vi "InvPendSfbTrking_277.vi"() -> ()   [LabVIEW 2016]
uses:
  <vilib>/Analysis/Matrix/Datatypes/RealMatrix.ctl
  <vilib>/Simulation/Scripting/Companion Diagram/SimConfigNode/SimParams.ctl
  <vilib>/Simulation/Scripting/Companion Diagram/SimConfigNode/_simSolvers.ctl
  <vilib>/Simulation/Implementation/Shared/SIMSCR Execution Mode.ctl
  <vilib>/Platform/TimedLoop/XDataNode/timing_clust.ctl
  <vilib>/Platform/TimedLoop/XDataNode/nitl_modes.ctl
  <vilib>/Platform/TimedLoop/XDataNode/wakeup.ctl
  <vilib>/Simulation/Param Hierarchy/Typedefs/SIMPH Param Control Actions.ctl
  <vilib>/Simulation/Implementation/Shared/NILVSim_ParamChanged.vi
  <vilib>/Simulation/Implementation/Shared/NILVSim_FinishedLate.vi
  <vilib>/Simulation/Implementation/Shared/NILVSIM_BeginStep.vi
  <vilib>/Simulation/Utility/Implementation/NILVSim Collector.llb/SIM Collector (scalar).vi
  <vilib>/Simulation/Utility/Implementation/SIM Halt.vi
  <vilib>/Simulation/DataSources/Implementation/NILVSim Sine Wave.llb/SIM Sine Wave (scalar).vi
  <vilib>/Simulation/DiscreteLinear/Implementation/NILVSim Discrete State Space Buffered.llb/SIM Discrete State Space Distributor (SISO).vi
  <vilib>/Simulation/DiscreteLinear/Implementation/NILVSim Discrete State Space Buffered.llb/SIM Discrete State Space Collector (SISO).vi
  <vilib>/Analysis/baseanly.llb/A x B.vi
  <vilib>/Analysis/baseanly.llb/A x Vector.vi
  <vilib>/Simulation/DiscreteLinear/Implementation/NILVSim Discrete Delay.llb/NILVSim Discrete Delay Buffered Distributor (vector).vi
  <vilib>/Simulation/Nonlinear/Implementation/NILVSim Saturation.llb/SIM Saturation (scalar).vi
  <vilib>/Simulation/DiscreteLinear/Implementation/NILVSim Discrete Delay.llb/NILVSim Discrete Delay Buffered Collector (vector).vi
  <vilib>/Simulation/Implementation/Shared/NILVSim_Manager.vi
  <vilib>/Utility/error.llb/Clear Errors.vi
  <vilib>/Simulation/Implementation/Shared/NILVSim_FinalizeModel.vi
  <vilib>/Simulation/Utility/Implementation/NILVSim Collector.llb/NILVSim Collector core (scalar).vi
  <vilib>/Simulation/Implementation/Shared/SIM Unbundle Sim Info.vi
  <vilib>/Simulation/Implementation/Shared/SIMSH Read Queue.vi
  <vilib>/Simulation/Implementation/Shared/NILVSim_Initialize.vi
  <vilib>/Simulation/Utility/Implementation/NILVSim Get Time and IsAcceptedStep.vi
  SubVI/CommandDuty.vi
  <vilib>/Simulation/Implementation/Shared/NILVSim_GetModelError.vi
  <vilib>/Simulation/Implementation/Shared/SIM Bundle Sim Info.vi
  <vilib>/Simulation/Scripting/Companion Diagram/SimConfigNode/SimDog.xnode
  <vilib>/Platform/TimedLoop/XDataNode/XDataNode.xnode
  <vilib>/Simulation/Implementation/XNodeFramework/SimXNode/SimX.xnode
  <vilib>/Analysis/NI_AALBase.lvlib
  <vilib>/Simulation/DiscreteLinear/Implementation/NILVSim Discrete Delay.llb/SIM Discrete Delay Buffered (vector).vi
  <vilib>/Simulation/DiscreteLinear/Implementation/NILVSim Discrete State Space Buffered.llb/SIM Discrete State Space Buffered (SISO).vi
  <vilib>/Platform/TimedLoop/XDataNode/XDNodeRunTimeDep.lvlib
  <vilib>/Simulation/Implementation/Shared/NI_SIM_Implementation.lvlib
  <vilib>/Analysis/Matrix/NI_Matrix.lvlib
panel:
  in  "Tab Control":T1(tab)
  out "Reference r and Output y":cluster{dbl, dbl}(graph)
  out "Control input u":dbl(graph)
  in  "Final Time (s)":dbl=10.0
  in  "Run Control":bool
  in  "K":T2=[[4.67, 70.57]]
  out "y_hat vs y":cluster{"Result":dbl, dbl}(graph)
  in  "Pc":T2=[[0.0, 2.15]]
  in  "Pa":T2=[[1.0012, 0.0117], [0.016, 1.0001]]
  in  "Pb":dbl[](array[numeric])=[0.1281, 0.0001]
  in  "L":dbl[](array[numeric])=[2.925, 0.279]
  in  "Km":T2=[[4.67, 70.57]]
  out "error out":errorcluster
  out "Counter Value":i32
  # "Control Settings"
  # "InvPend Model"
  # "Control Parameters"
  # "Hint: You don't need to do anything in this page"
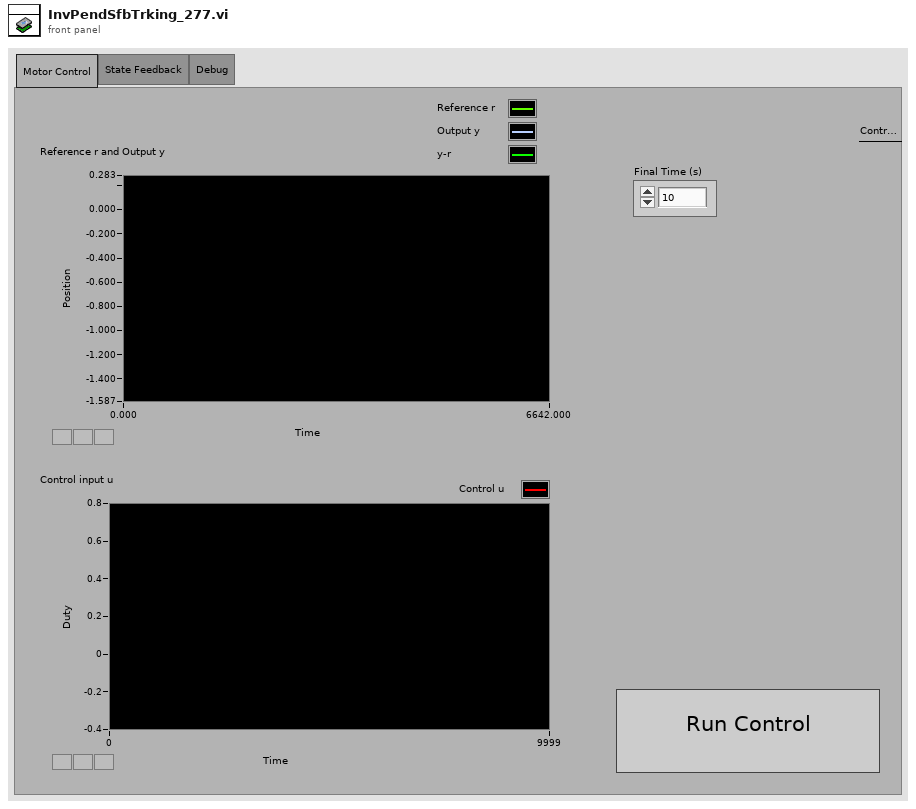
[diagram p1: front panel]
types:
  T1 = enum32{"Motor Control", "State Feedback", "Debug"}
  T2 = typedef "NI_Matrix.lvlib/RealMatrix.ctl" = dbl[][]
  T3 = typedef "SIMSCR Execution Mode.ctl" = enum16{"Simulate to Completion", "Single Time-Step Simulation (Fixed Step Only)"}
  T4 = typedef "XDNodeRunTimeDep.lvlib/timing_clust.ctl" = cluster{"Expected End [f-1]":u64, "Actual End [f-1]":u64, "Finished Late? [f-1]":bool, "Expected End [i-1]":u64, "Actual End [i-1]":u64, "Finished Late? [i-1]":bool, "Expected Start [i]":u64, "Actual Start [i]":u64, "Expected Start [f]":u64, "Actual Start [f]":u64, "Source Name":string, "Structure Name":string, "Period":i64, "Deadline":i64, "Offset":i64, "Start":i64, "Priority":i32, "Timeout":i32, "Mode":T5, "Wakeup Reason":T6, "Error":errorcluster, "Source Type":string, "Secondary Source Type":string, "Global End Time":u64, "Global Start Time":u64, "Frame Duration":u64, "Iteration Duration":u64, "Assigned CPU":i32, "I/O Scan Engine Mode":u32}
  T5 = typedef "XDNodeRunTimeDep.lvlib/nitl_modes.ctl" = enum32{"No Change", "Process missed periods, maintain original phase", "Discard missed periods, maintain original phase", "Process missed periods, ignore original phase", "Discard missed periods, ignore original phase"}
  T6 = typedef "XDNodeRunTimeDep.lvlib/wakeup.ctl" = enum32{"Normal", "Aborted", "Asynchronous wakeup", "Timing source error", "Timed loop error", "Timeout"}
  T7 = typedef "SIMPH Param Control Actions.ctl" = enum16{"get params", "set params"}
  T8 = typedef "SimParams.ctl" = cluster{"Initial Time (s)":dbl, "Final Time (s)":dbl, "Step Size (s)":dbl, "ODE Solver":T9, "Minimum Step Size (s)":dbl, "Maximum Step Size (s)":dbl, "Relative Tolerance":dbl, "Absolute Tolerance":dbl, "Software Timing":bool, "Initial Step Size (s)":dbl, "Automatic Fixed Step Size?":bool, "Automatic Discrete Step Size?":bool, "Discrete Step Size (s)":dbl, "Calculate using Time Step":bool, "Solver Wired?":bool, "Prev.Frm.Expected End":u64, "Prev.Frm.Actual End":u64, "Prev.Frm.Finished Late?":bool, "Prev.Iter.Expected End":u64, "Prev.Iter.Actual End":u64, "Prev.Iter.Finished Late?":bool, "Expected Iteration Start":u64, "Actual Iteration Start":u64, "Expected Frame Start":u64, "Actual Frame Start":u64, "Source Name":string, "Name":string, "Period":i64, "Deadline":i64, "Offset":i64, "Start":i64, "Priority":i32, "Timeout":i32, "Processor":i32, "Mode":enum32{"No Change", "Process missed periods, maintain original phase", "Discard missed periods, maintain original phase", "Process missed periods, ignore original phase", "Discard missed periods, ignore original phase"}, "Wakeup reason":enum32{"Normal", "Aborted", "Asynchronous wakeup", "Timing source error", "Timed loop error", "Timeout"}, "Error":errorcluster, "Source Type":string, "Secondary Source Type":string, "Global End Time":u64, "Global Start Time":u64, "Full Solver Reset":bool, "Execution Mode":T3, "Nan/Inf Check":bool, "Custom Solver Library":string, "Solver Is Variable":bool, "custom solver name":string, "Signal Collection Decimation":u32}
  T9 = typedef "_simSolvers.ctl" = enum16{"Runge-Kutta 1 (Euler)", "Runge-Kutta 2", "Runge-Kutta 3", "Runge-Kutta 4", "Runge-Kutta 23 (variable)", "Runge-Kutta 45 (variable)", "BDF (variable)", "Adams-Moulton (variable)", "Rosenbrock (variable)", "Discrete States Only", "SDIRK 4 (variable)", "Radau 5 (variable)", "Radau 9 (variable)", "Radau 13 (variable)", "Radau [Variable Order] (variable)", "Gear's Method (variable)", "Linearizer", "State Query", "Trim Eval", "Custom Solver"}
  T10 = typedef "PWM.lvlib/PWM Reference.ctl" = cluster{"myRIO Reference":T11, "PWM Channels Enum":T15, "PWM Configuration":T16}
  T11 = typedef "myRIO Generic Hardware Reference.ctl" = cluster{"myRIO Model":T12, "myRIO Hardware Reference":T13}
  T12 = typedef "Hardware Version Enum.ctl" = enum16{"Unknown", "myRIO-1900", "myRIO-1950", "roboRIO", "NI ELVIS RIO CM"}
  T13 = typedef "myRIO v1.0 Reference.ctl" = cluster{"Generic FPGA Reference":T14, "Allow multiple opens":bool}
  T14 = typedef "Generic FPGA Reference.ctl" = refnum<k20>
  T15 = typedef "PWM Channels Enum.ctl" = enum16{"Not Connected", "C/PWM0", "C/PWM1", "A/PWM0", "A/PWM1", "A/PWM2", "B/PWM0", "B/PWM1", "B/PWM2", "PWM/PWM0", "PWM/PWM1", "PWM/PWM2", "PWM/PWM3", "PWM/PWM4", "PWM/PWM5", "PWM/PWM6", "PWM/PWM7", "PWM/PWM8", "PWM/PWM9"}
  T16 = typedef "PWM.lvlib/PWM Configuration.ctl" = cluster{"Frequency":dbl, "Duty Cycle":dbl}
  T17 = typedef "Encoder.lvlib/Encoder Reference.ctl" = cluster{"myRIO Reference":T11, "Encoder Channels Enum":T18}
  T18 = typedef "Encoder Channels Enum.ctl" = enum16{"Not Connected", "C/ENC0", "C/ENC1", "A/ENC", "B/ENC", "DIO/ENC0", "DIO/ENC1", "DIO/ENC2", "DIO/ENC3", "DIO/ENC4"}
  T19 = typedef "DIO.lvlib/DIO Reference.ctl" = cluster{"myRIO Reference":T11, "DIO Channels List":T20}
  T20 = typedef "DIO Channels List.ctl" = T21[]
  T21 = typedef "DIO Channels Enum.ctl" = enum16{"Not Connected", "C/DIO0", "C/DIO1", "C/DIO2", "C/DIO3", "C/DIO4", "C/DIO5", "C/DIO6", "C/DIO7", "A/DIO0", "A/DIO1", "A/DIO2", "A/DIO3", "A/DIO4", "A/DIO5", "A/DIO6", "A/DIO7", "A/DIO8", "A/DIO9", "A/DIO10", "A/DIO11", "A/DIO12", "A/DIO13", "A/DIO14", "A/DIO15", "B/DIO0", "B/DIO1", "B/DIO2", "B/DIO3", "B/DIO4", "B/DIO5", "B/DIO6", "B/DIO7", "B/DIO8", "B/DIO9", "B/DIO10", "B/DIO11", "B/DIO12", "B/DIO13", "B/DIO14", "B/DIO15", "LED0", "LED1", "LED2", "LED3", "Button0", "DIO/DIO0", "DIO/DIO1", "DIO/DIO2", "DIO/DIO3", "DIO/DIO4", "DIO/DIO5", "DIO/DIO6", "DIO/DIO7", "DIO/DIO8", "DIO/DIO9", "SPI/CS0", "SPI/CS1", "SPI/CS2", "SPI/CS3", "LED RADIO (Green)", "LED RADIO (Red)", "LED COMM (Green)", "LED COMM (Red)", "LED MODE (Green)", "LED MODE (Red)"}
  T22 = cluster{"PWM0":T10, "PWM1":T10, "Encoder":T17, "En":T19}
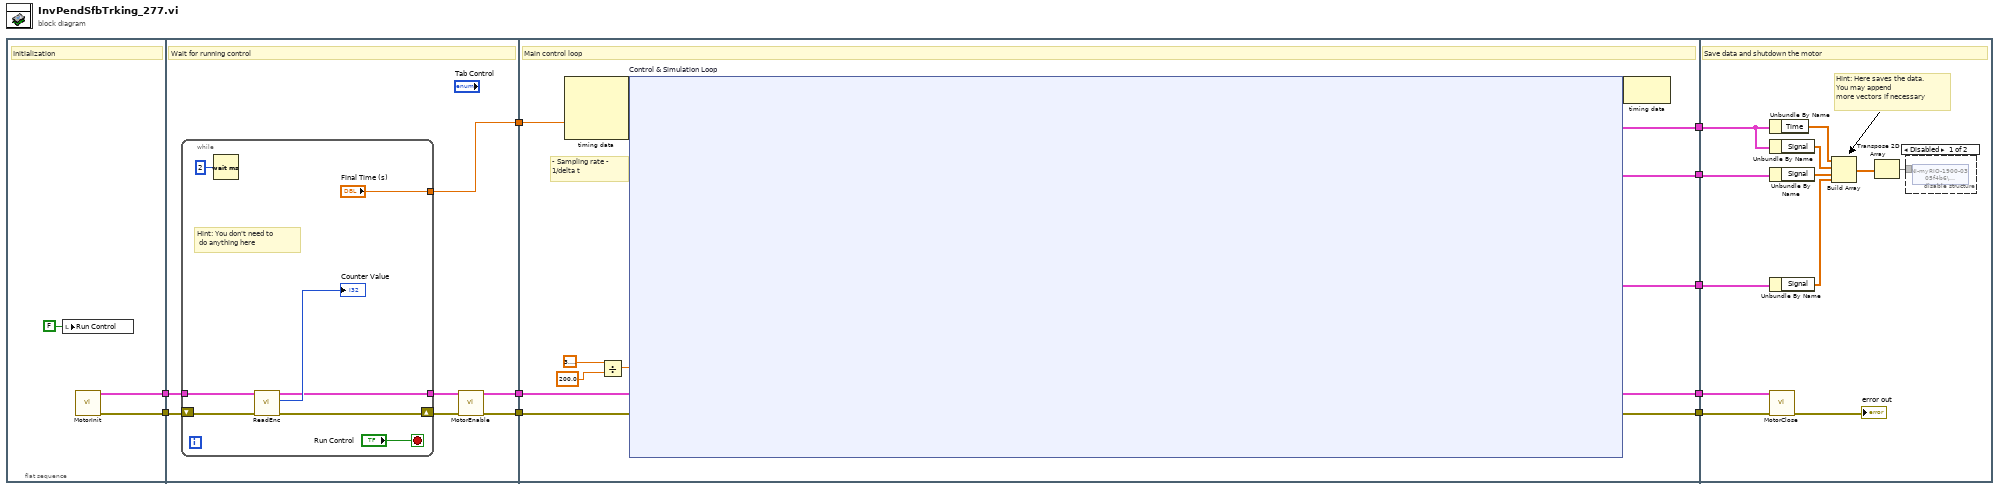
[diagram p0: block diagram]
diagram:
  n1 = flat-sequence {
    tunnel: [w12] -> w2
    tunnel: [w11] -> w1
    tunnel: [w14] -> w10
    tunnel: [w16] -> w9
    tunnel: [w15] -> w4
    tunnel: w2 -> [w20]
    tunnel: w1 -> [w19]
    tunnel: w10 -> [w38]
    tunnel: w9 -> [w37]
    tunnel: [w36] -> w8
    tunnel: [w35] -> w7
    tunnel: [w34] -> w6
    tunnel: [w33] -> w5
    tunnel: w4 -> [w39]
    tunnel: [w32] -> w3
    tunnel: w8 -> [w644]
    tunnel: w7 -> [w643]
    tunnel: w6 -> [w642]
    tunnel: w5 -> [w641]
    tunnel: w3 -> [w639]
    frame #0 {
      # "Initialization"
      n2 = local write "Run Control"(FALSE ("Run Control")) -> ()
      n3 = call "MotorInit.vi"() -> ("error out"=w11:errorcluster, "Cluster"=w12:T22)  [unwired: 10 in]
    }
    frame #1 {
      # "Wait for running control"
      n4 = while {
        tunnel: w20 -> [w24]
        tunnel: [w23] -> w18
        shift-right: [w22] -> w17
        shift-left: w19 -> [w26]
        tunnel: ["Final Time (s)"] -> w14
        stop <- "Run Control" stop-if-true
        # "Hint: You don't need to\n do anything here"
        n5 = Wait (ms)(milliseconds to wait=u32 2) -> ()  [unwired: 1 out]
        n6 = call "ReadEnc.vi"("error in"=w26, "Cluster In"=w24) -> ("error out"=w22:errorcluster, "Enc value [count]"=→"Counter Value":i32, "Cluster Out"=w23:T22)  [unwired: 7 in]
      }
      n7 = call "MotorEnable.vi"("error in"=w17, "Cluster In"=w18) -> ("error out"=w16:errorcluster, "Cluster Out"=w15:T22)  [unwired: 8 in]
    }
    frame #2 {
      # "- Sampling rate -\n1/delta t"
      # "Main control loop"
      n8 = node-c288(w38) -> (w41:variant)  [unwired: 3 in]
      n9 = Divide(x=3.141592653589793, y=200.0) -> (x/y=w31:dbl)
      n10 = node-c254 "Control & Simulation Loop"(w41, w39, w37, w31) -> (w40:variant, w36:cluster{"Time":dbl[], "Signal":dbl[]}, w35:cluster{"Time":dbl[], "Signal":dbl[]}, w33:errorcluster, w34:T22, w32:cluster{"Time":dbl[], "Signal":dbl[]})
      n11 = node-c288(w40) -> ()  [unwired: 1 out]
    }
    frame #3 {
      # "Hint: Here saves the data.\nYou may append\nmore vectors if necessary"
      # "Save data and shutdown the motor"
      n12 = Unbundle By Name(w639) -> ("Time"=w638:dbl[])
      n13 = Unbundle By Name(w639) -> ("Signal"=w637:dbl[])
      n14 = Unbundle By Name(w644) -> ("Signal"=w636:dbl[])
      n15 = Unbundle By Name(w643) -> ("Signal"=w635:dbl[])
      n16 = call "MotorClose.vi"("error in (no error)"=w641, "Cluster"=w642) -> ("error out"=→"error out":errorcluster)  [unwired: 9 in]
      n17 = Build Array(w638, w637, w636, w635) -> (w634:dbl[][])
      n18 = Transpose 2D Array(2D array=w634) -> (transposed array=w633:dbl[][])
      n19 = disable-structure shown="Disabled" {
        disable-tunnel: w633 -> [w645 _]
        frame Disabled {
          n20 = shared-variable "NI-myRIO-1900-0305f4b6\\MyVariables.lvlib\\Data"(w645) -> ()  [unwired: 1 in, 1 out]
        }
        frame Enabled {
        }
      }
    }
  }
